vi "HSPA_QAM_Rx.vi"() -> ()   [LabVIEW 2025]
uses:
  <vilib>/addons/Modulation/Analog/support/mod_Set Error Source.vi
  <vilib>/addons/Modulation/Digital/Support/Common/Validators/mod_Generate Filter Coefficients Validate.vi
  <vilib>/addons/Modulation/Digital/General/subVIs/mod_Generate Filter Coefficients.vi
  <vilib>/addons/Modulation/Digital/General/MT Generate QAM System Parameters(M).vi
  <instrlib>/niUSRP/niUSRP Fetch Rx Data (CDB Cluster).vi
  <vilib>/addons/Modulation/niDMT.lvlib
panel:
  in  "stop 2":bool
  in  "samples per symbol (16)":i32=16
  in  "matched samples per symbol (16)":i32=16
  out "Constellation Graph":T1(graph)
  in  "pulse shaping samples per symbol (16)":i32=16
  in  "pulse shaping filter (none)":T2(ring)
  out "coerced gain":dbl format="%#_6f"
  out "coerced carrier frequency":dbl=100000.0 format="%#_6p"
  out "coerced IQ rate":dbl=100000.0 format="%#_6p"
  in  "Recv carrier frequency":dbl=100000.0 format="%#_6p"
  in  "Recv IQ rate":dbl=100000.0 format="%#_6p"
  in  "number of samples":i64=100000
  in  "active antenna 2":string
  in  "gain":dbl format="%#_6f"
  out "error out":errorcluster
  in  "error in (no error)":errorcluster
  in  "USRP IP Address":refnum<k15>
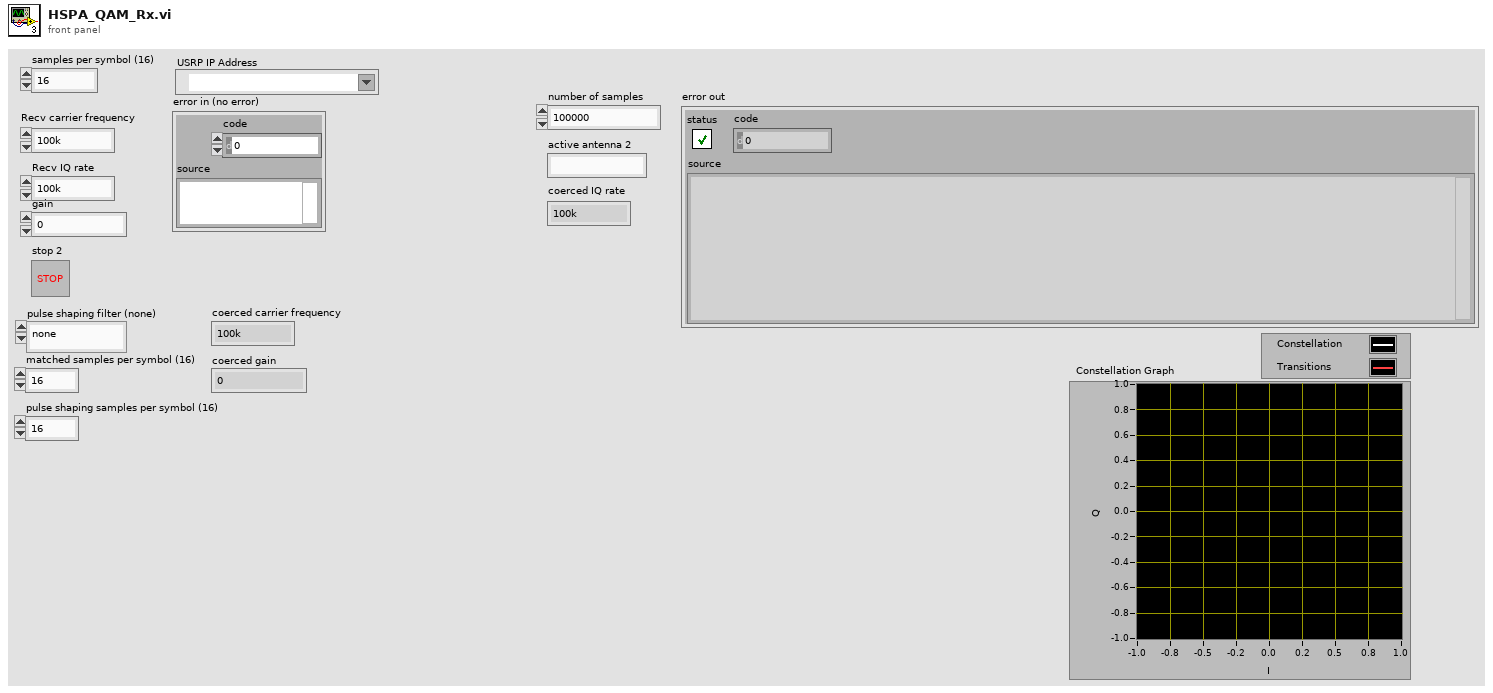
[diagram p1: front panel]
types:
  T1 = cluster{"Decimated Array":dbl[], "Decimated Array":dbl[]}[]
  T2 = enum16{"none", "Raised Cosine", "Root Raised Cos", "Gaussian"}
  T3 = enum16{"FSK", "PSK", "QAM", "MSK", "PAM", "ASK", "CPM"}
  T4 = cluster{"samples per symbol (16)":i32, "symbol map":cdb[]}
  T5 = typedef "niAMT.lvlib/Complex Data Waveform.ctl" = cluster{"t0":dbl, "dt":dbl, "Y":cdb[]}
  T6 = cluster{"constellation":dbl[], "oversampled data":dbl[]}[]
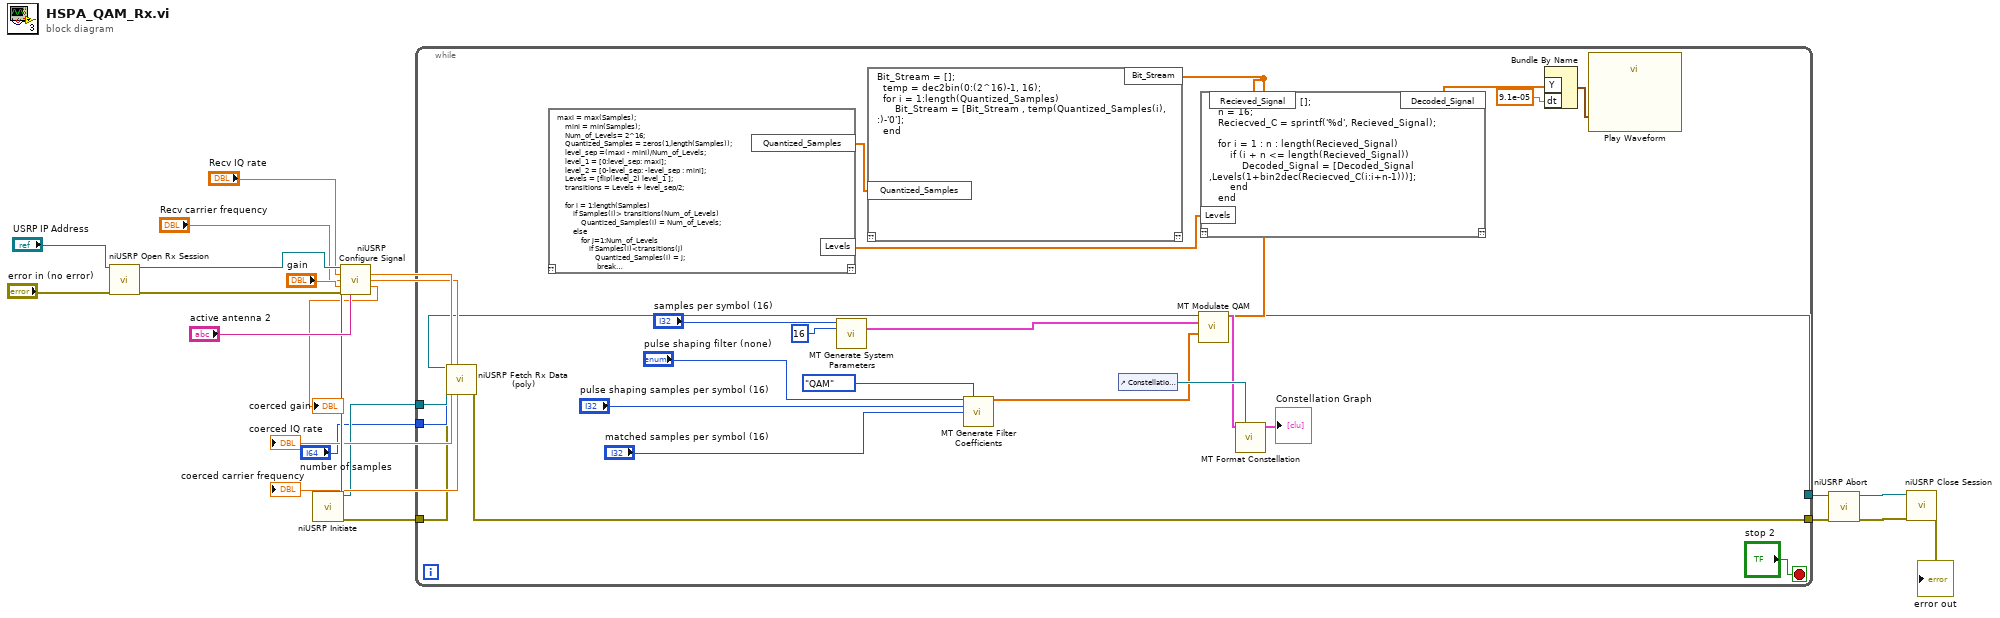
[diagram p0: block diagram]
diagram:
  n1 = call <instrlib>:"niUSRP Open Rx Session.vi"("device names"="USRP IP Address", "error in (no error)"="error in (no error)") -> ("session handle out"=w19:refnum<k15>, "error out"=w18:errorcluster)  [unwired: 12 in]
  n2 = call <instrlib>:"niUSRP Configure Signal.vi"("session handle"=w19, "IQ rate"="Recv IQ rate", "carrier frequency"="Recv carrier frequency", "gain"="gain", "error in (no error)"=w18, "active antenna"="active antenna 2") -> ("session handle out"=w15:refnum<k15>, "coerced IQ rate"=→"coerced IQ rate":dbl, "coerced carrier frequency"=→"coerced carrier frequency":dbl, "coerced gain"=→"coerced gain":dbl, "error out"=w14:errorcluster)  [unwired: 5 in]
  n3 = call <instrlib>:"niUSRP Initiate.vi"("session handle"=w15, "error in (no error)"=w14) -> ("session handle out"=w5:refnum<k15>, "error out"=w3:errorcluster)  [unwired: 12 in]
  n4 = while {
    tunnel: w5 -> [w26]
    tunnel: "number of samples" -> [w25]
    tunnel: w3 -> [w24]
    tunnel: [w23] -> w2
    tunnel: [w22] -> w1
    stop <- "stop 2" stop-if-true
    n5 = call-poly <instrlib>:"niUSRP Fetch Rx Data (poly).vi"("session handle"=w26, "number of samples"=w25, "error in (no error)"=w24) -> ("session handle out"=w23:refnum<k15>, "error out"=w22:errorcluster)  [unwired: 9 in, 2 out]
    n6 = script code="maxi = max(Samples);\n    mini = min(Samples);\n    Num_of_Levels= 2^16;\n    Quantized_Samples = zeros(1,length(Samples));\n    level_sep =(maxi - mini)/Num_of_Levels; \n    level_1 = [0:level_sep: maxi];\n    level_2 = [0-level_sep: -level_sep : mini];\n    Levels = [flip(level_2) level_1 ];\n    transitions = Levels + level_sep/2;\n    \n    for i = 1:length(Samples)\n        if Samples(i)> transitions(Num_of_Levels)\n            Quantized_Samples(i) = Num_of_Levels;\n        else\n            for j=1:Num_of_Levels\n                if Samples(i)<transitions(j)\n                   Quantized_Samples(i) = j;\n                    break\n                end\n            end\n        end\n    end"() -> ("Quantized_Samples"=w35:dbl[], "Levels"=w36:dbl[])  [unwired: 1 in, 1 out]
    n7 = call-poly <vilib>:"MT Generate System Parameters.vi"("samples per symbol (16)"="samples per symbol (16)", "M-QAM (16)"=16 ("M-PSK (4)")) -> ("QAM system parameters"=w29:T4)  [unwired: 11 in, 2 out]
    n8 = script code="Bit_Stream = [];\n  temp = dec2bin(0:(2^16)-1, 16);  \n  for i = 1:length(Quantized_Samples)\n      Bit_Stream = [Bit_Stream , temp(Quantized_Samples(i), :)-'0'];\n  end"("Quantized_Samples"=w35) -> ("Bit_Stream"=w27:dbl[])  [unwired: 1 in, 1 out]
    n9 = call <vilib>:"MT Generate Filter Coefficients.vi"("pulse shaping filter (none)"="pulse shaping filter (none)", "modulation type"=T3."QAM", "pulse shaping samples per symbol (16)"="pulse shaping samples per symbol (16)", "matched samples per symbol (16)"="matched samples per symbol (16)") -> ("pulse shaping filter coefficients"=w28:dbl[])  [unwired: 9 in, 2 out]
    n10 = control-ref of="Constellation Graph"() -> (w42:refnum<vi>)
    n11 = call <vilib>:"MT Modulate QAM.vi"("input bit stream"=w27, "QAM system parameters"=w29, "pulse shaping filter coefficients"=w28) -> ("output complex waveform"=w30:T5)  [unwired: 10 in, 2 out]
    n12 = script code="Decoded_Signal = [];\n   n = 16;\n   Reciecved_C = sprintf('%d', Recieved_Signal);\n   \n   for i = 1 : n : length(Recieved_Signal)\n       if (i + n <= length(Recieved_Signal))\n           Decoded_Signal = [Decoded_Signal ,Levels(1+bin2dec(Reciecved_C(i:i+n-1)))];\n       end\n   end"("Recieved_Signal"=w27, "Levels"=w36) -> ("Decoded_Signal"=w34:dbl[])  [unwired: 1 in, 1 out]
    n13 = call <vilib>:"MT Format Constellation.vi"("waveform"=w30, "constellation reference"=w42) -> ("constellation graph"=→"Constellation Graph":T6)  [unwired: 3 in, 10 out]
    n14 = Bundle By Name("Y"=w34, "dt"=9.1e-05) -> (w33:waveform(dbl))  [unwired: 1 in]
    n15 = call "Play Waveform"("Data"=w33) -> ()  [unwired: 18 in, 1 out]
  }
  n16 = call <instrlib>:"niUSRP Abort.vi"("session handle"=w2, "error in (no error)"=w1) -> ("session handle out"=w13:refnum<k15>, "error out"=w12:errorcluster)  [unwired: 12 in]
  n17 = call <instrlib>:"niUSRP Close Session.vi"("session handle"=w13, "error in (no error)"=w12) -> ("error out"=→"error out":errorcluster)  [unwired: 13 in]
